vi "ProgressBar-Bundle data.vi"(8 "Sender":enum16{"Acquisition", "Logging", "File gen"}(ring), 9 "Message in":string, 10 "Current":i32, 11 "Total":i32) -> (2 "Progress bar window values input":T1)   [LabVIEW 2020]
uses:
  Progress bar window values input cluster.ctl
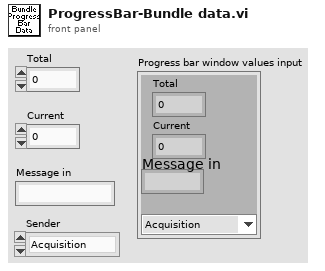
[diagram p1: front panel]
types:
  T1 = typedef "Progress bar window values input cluster.ctl" = cluster{"Total":i32, "Current":i32, "Message in":string, "Sender":enum16{"Acquisition", "Logging", "File gen"}}
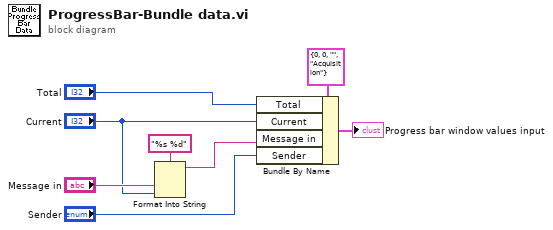
[diagram p0: block diagram]
diagram:
  n1 = Format Into String(format string="%s %d", "Message in", "Current") -> (resulting string=w5:string)  [unwired: 2 in, 1 out]
  n2 = Bundle By Name(cluster=T1 {"Total"=0, "Current"=0, "Message in"="", "Sender"=enum."Acquisition"} ("Progress bar window values input"), "Total"="Total", "Current"="Current", "Message in"=w5, "Sender"="Sender") -> (→"Progress bar window values input":T1)
